vi "Toolbar Index Button.vi"(7 "error In (no error)":errorcluster, 8 "Index":variant, 9 "Container State":T1, 10 "Display State In":T2={"Buttons Displayed"=0, "Button States"=[], "Button Size"=0, "Button Style"=enum."Classic", "Active Button"=0, "Force Regen?"=FALSE, "Tip String Ref"=refnum}) -> (0 "error out":errorcluster, 3 "Output":refnum<class "Button.lvclass">[](array[class]), 4 "index of element":i32)   [LabVIEW 2012, in "Toolbar.xctl"]
doc: "Indexes the array of buttons either as a number (with bounds cjhecking) or as a string by looking for an exact match with the button name. Uses the state information to collect the list of buttons from the volatile state store."
uses:
  Toolbar.xctl
  Button_Class/Button.lvclass
  Toolbar State.ctl
  Button_Class/Type Defs/Button Style.ctl
  <vilib>/_xctls/Container State.ctl
  <vilib>/Utility/VariantDataType/VariantType.lvlib
  <vilib>/_xctls/XControlSupport.lvlib
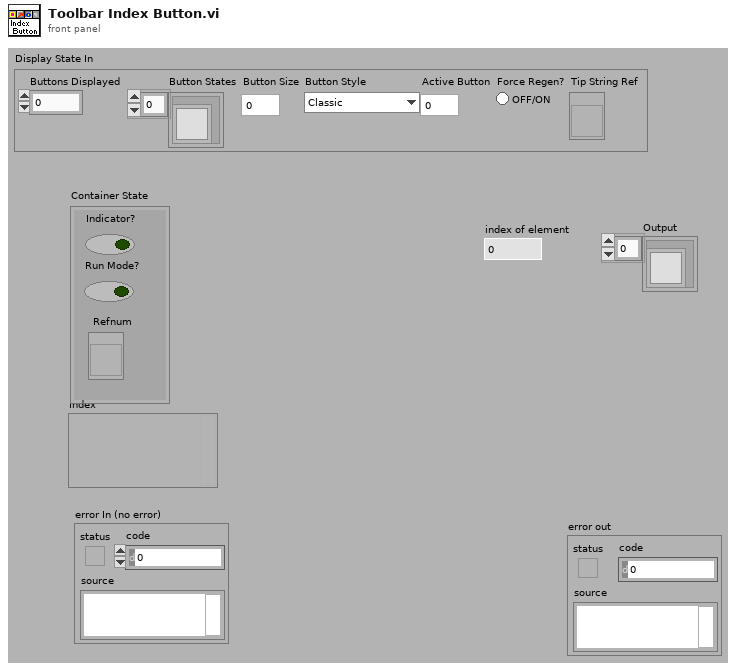
[diagram p1: front panel]
types:
  T1 = typedef "XControlSupport.lvlib/Container State.ctl" = cluster{"Indicator?":bool, "Run Mode?":bool, " Refnum":refnum<vi>}
  T2 = typedef "Toolbar.xctl/Toolbar State.ctl" = cluster{"Buttons Displayed":i32, "Button States":refnum<class "Button.lvclass">[], "Button Size":i32, "Button Style":T3, "Active Button":i32, "Force Regen?":bool, "Tip String Ref":refnum<vi>}
  T3 = typedef "Button.lvclass/Button Style.ctl" = enum16{"System", "Modern", "Classic", "Rounded", "Silver", "Ni Theme", "Metallic"}
  T4 = typedef "VariantType.lvlib/Type.ctl" = enum8{"Invalid Type", "Void", "I8", "I16", "I32", "I64", "U8", "U16", "U32", "U64", "Single Float", "Double Float", "Extended Float", "Single Complex", "Double Complex", "Extended Complex", "Enum U8", "Enum U16", "Enum U32", "Enum U64", "Single Float With Unit", "Double Float With Unit", "Extended Float With Unit", "Single Complex with Unit", "Double Complex with Unit", "Extended Complex with Unit", "Boolean", "String", "Path", "Picture", "Tag", "Array", "Cluster", "Variant", "LV Variant", "Waveform", "Timestamp", "Digital Waveform", "Digital Data", "ExpressData", "Refnum", "External Data", "VI", "Poly VI", "LabVIEW Class Instance", "Fixed Point"}
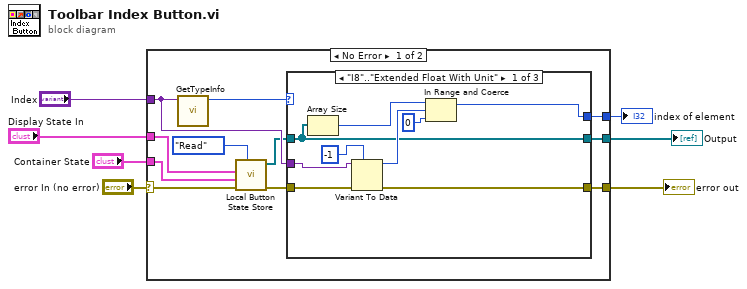
[diagram p0: block diagram]
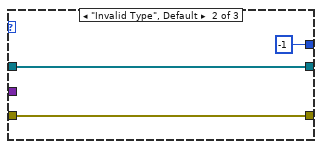
[diagram p2: hidden frame]
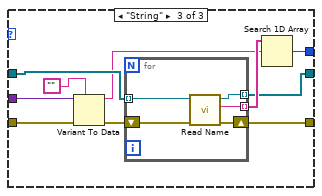
[diagram p3: hidden frame]
diagram:
  n1 = case shown="No Error" "error In (no error)" {
    selector: "error In (no error)" -> [w13 w46]
    tunnel: [w18 w46] -> w7
    tunnel: [w17 _] -> w6
    tunnel: [w16 _] -> w5
    tunnel: "Index" -> [w15 _]
    tunnel: "Display State In" -> [w9 _]
    tunnel: "Container State" -> [w8 _]
    frame No Error {
      n2 = call <vilib>:"GetTypeInfo.vi"("Variant"=w15) -> ("Type Enum"=w11:T4)  [unwired: 1 in, 9 out]
      n3 = call "Local Button State Store.vi"("Operation"=enum16{"Read", "Write"}."Read", "error in (no error)"=w13, "Container State"=w8, "Display State In"=w9) -> ("error out"=w14:errorcluster, "Button States"=w12:refnum<class "Button.lvclass">[])  [unwired: 6 out]
      n4 = case shown="\"I8\"..\"Extended Float With Unit\"" w11 {
        tunnel: w12 -> [w20 w30 w38]
        tunnel: w14 -> [w25 w29 w37]
        tunnel: w15 -> [w27 _ w40]
        tunnel: [w22 -1 w33] -> w16
        tunnel: [w24 w29 w32] -> w18
        tunnel: [w20 w30 w31] -> w17
        frame "I8".."Extended Float With Unit" {
          n5 = Array Size(array=w20) -> (size(s)=w19:i32)
          n6 = Variant To Data(error in=w25, type=-1, Variant=w27) -> (data=w23:i32, error out=w24:errorcluster)
          n7 = In Range and Coerce(upper limit=w19, x=w23, lower limit=0 ("x")) -> (coerced(x)=w22:i32)  [unwired: 1 out]
        }
        frame "Invalid Type", Default {
        }
        frame "String" {
          n8 = Variant To Data(error in=w37, type="", Variant=w40) -> (data=w34:string, error out=w36:errorcluster)
          n9 = for {
            tunnel: w38 -> [w45] mode=indexing
            shift-right: [w43] -> w32
            shift-left: w36 -> [w44]
            tunnel: [w42] -> w35 mode=indexing
            tunnel: [w41] -> w31 mode=indexing
            n10 = call-dynamic "Read Name.vi"("error in (no error)"=w44, "Button.lvclass in"=w45) -> ("error out"=w43:errorcluster, "Name"=w42:string, "Button.lvclass out"=w41:refnum<class "Button.lvclass">)  [unwired: 7 out]
          }
          n11 = Search 1D Array(1D array=w35, element=w34) -> (index of element=w33:i32)  [unwired: 1 out]
        }
      }
    }
    frame Error {
    }
  }
  "error out" <- w7
  "Output" <- w6
  "index of element" <- w5
